vi "KeyboardSimCore.vi"(0 "VI Reference In":refnum<vi>, 1 "Label (VI Title)":string="Default", 11 "error in (no error)":errorcluster) -> (4 "VI Reference Out":refnum<vi>, 15 "error out":errorcluster)   [LabVIEW 2016, in "DronaTest.lvlib"]
uses:
  DronaTest.lvlib
  apis/Stimulus/KeyBoardSimulation/KeyBoardSimulation.vi
  APIs/Assert/AssertControlValue/Equal.vi
  <vilib>/addons/_JKI Toolkits/Caraya/classes/Assert/Assert Not Error.vi
  <vilib>/addons/_JKI Toolkits/Caraya/classes/Test/Test.lvclass
  Drona.lvlib
  <vilib>/addons/_JKI Toolkits/Caraya/classes/Assert/Assert.lvclass
  apis/Stimulus/KeyBoardSimulation/KeyboardSimulation.lvlib
  apis/Assert/AssertControlValue/AssertControlValue.lvlib
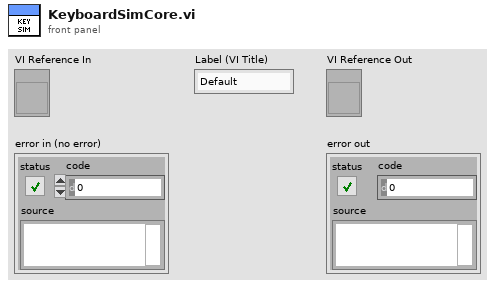
[diagram p1: front panel]
types:
  T1 = enum16{"Typing hello", "Paste from clipboard", "Numeric in range", "Numeric out of range positive", "Numeric out of range negative"}[]
  T2 = cluster{" Key":u8, "Action":enum16{"Press", "Up", "Down"}, "Delay (ms)":u32}[]
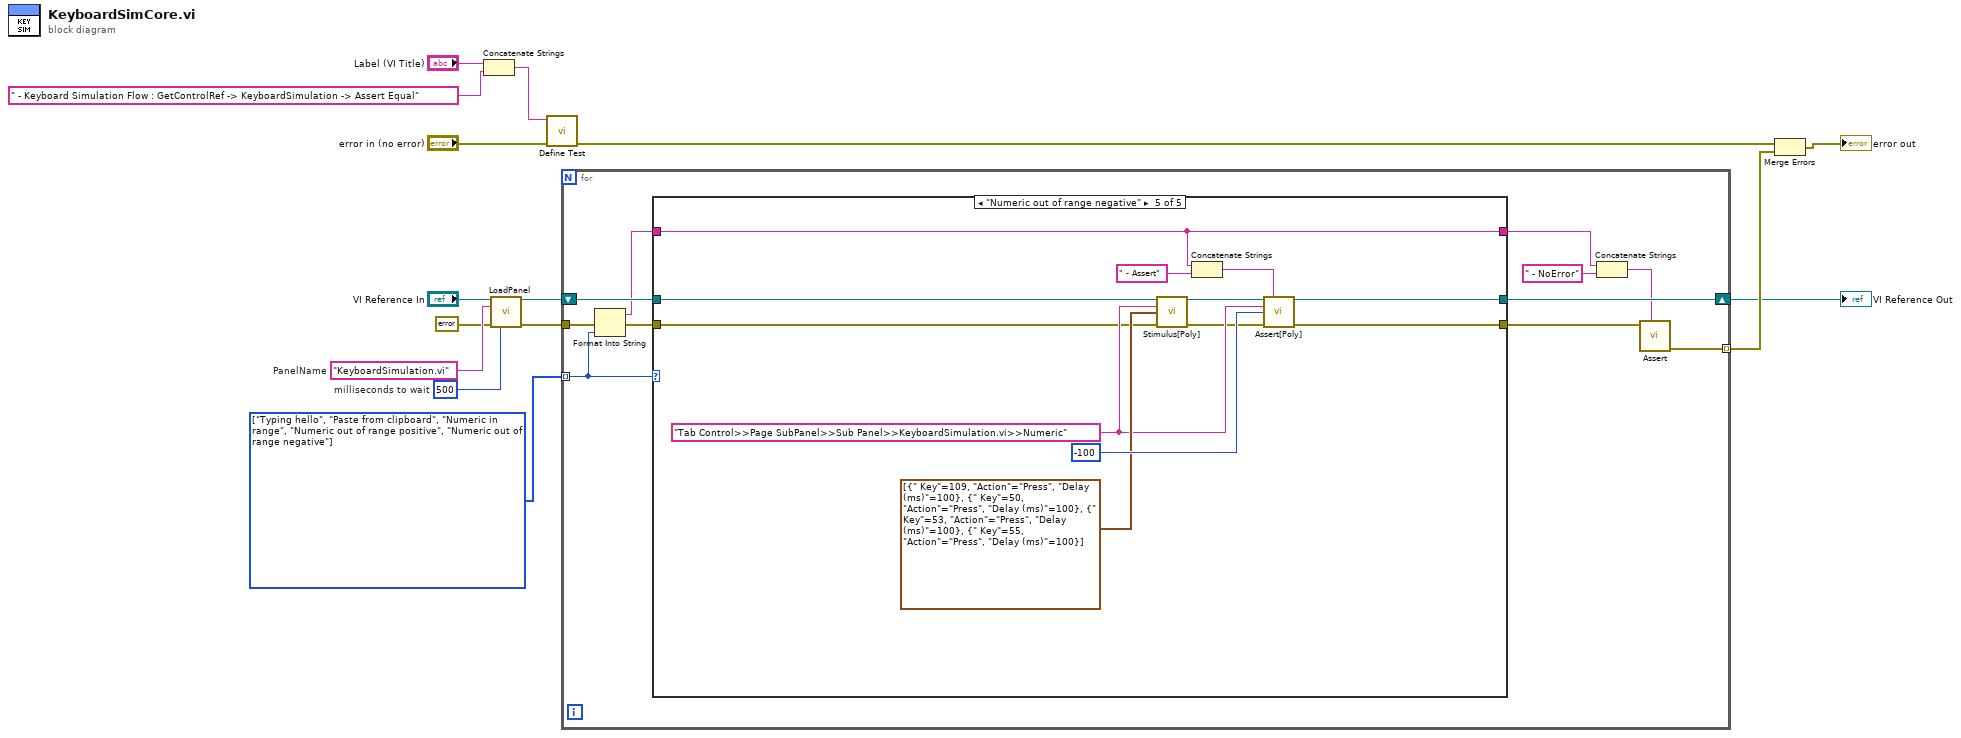
[diagram p0: block diagram]
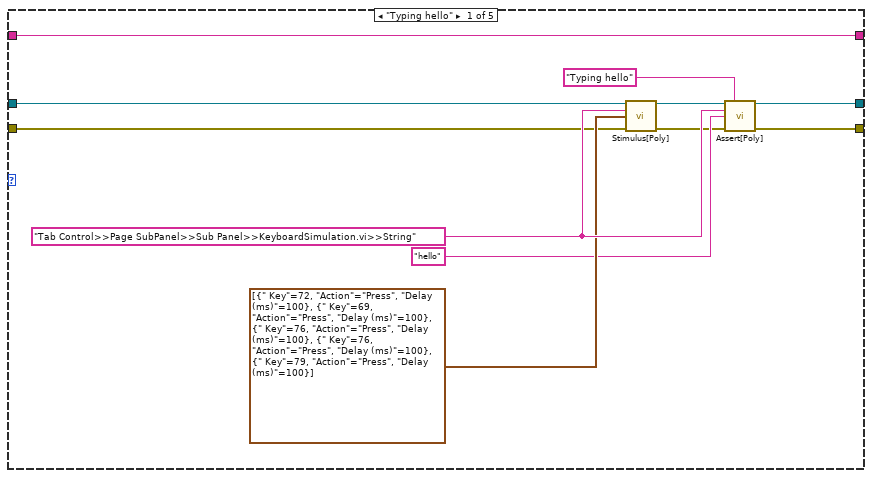
[diagram p2: hidden frame]
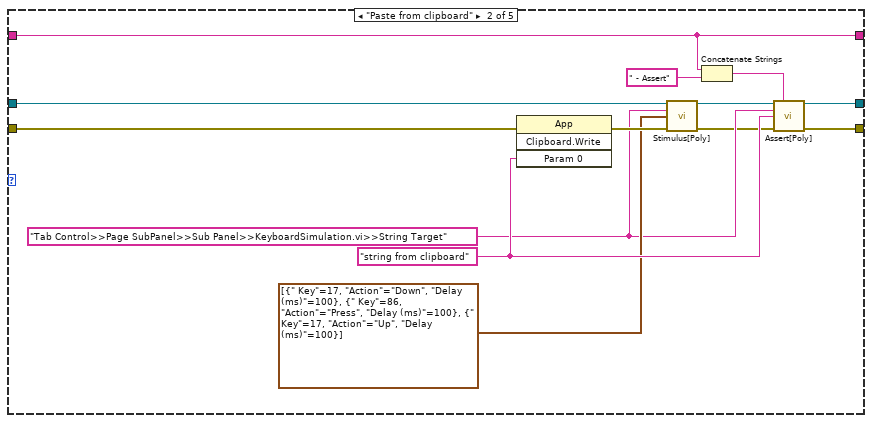
[diagram p3: hidden frame]
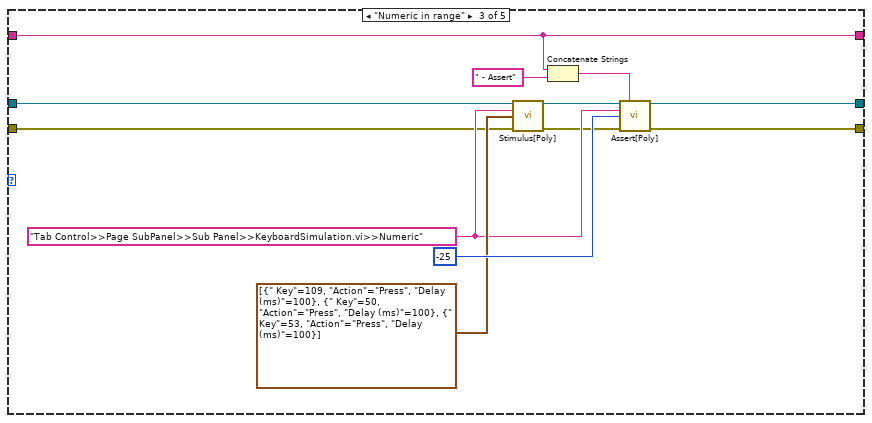
[diagram p4: hidden frame]
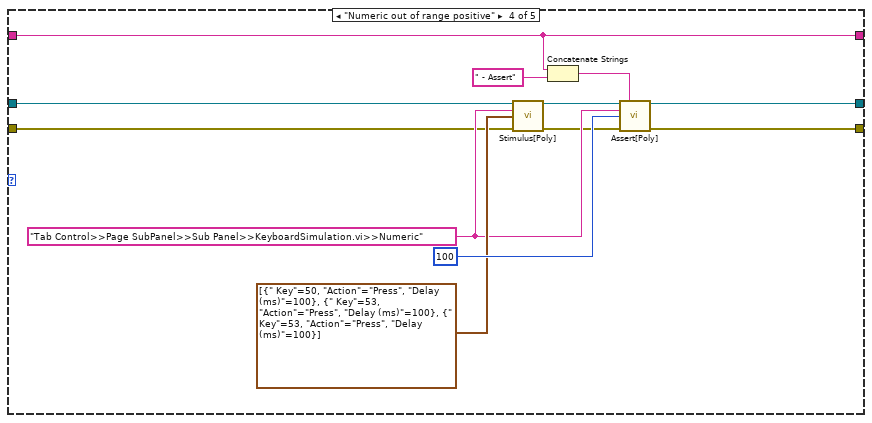
[diagram p5: hidden frame]
diagram:
  w5 = T1 [enum."Typing hello", enum."Paste from clipboard", enum."Numeric in range", enum."Numeric out of range positive", enum."Numeric out of range negative"] items=["Typing hello", "Paste from clipboard", "Numeric in range", "Numeric out of range positive", "Numeric out of range negative"] ("TestCases")
  w6 = u32 500  # milliseconds to wait
  w8 = "KeyboardSimulation.vi"  # PanelName
  n1 = Concatenate Strings("Label (VI Title)", " - Keyboard Simulation Flow : GetControlRef -> KeyboardSimulation -> Assert Equal" ("Label (VI Title)")) -> (w10:string)
  n2 = call "LoadPanel.vi"("VI in"="VI Reference In", "Panel Name"=w8, "error in (no error)"=errorcluster {"status"=FALSE, "code"=0, "source"=""} ("error in"), "milliseconds to wait"=w6) -> ("VI out"=w2:refnum<vi>, "error out"=w4:errorcluster)  [unwired: 10 in]
  n3 = call <vilib>:"Define Test.vi"("error in (no error)"="error in (no error)", "Label (VI Title)"=w10) -> ("error out"=w13:errorcluster)  [unwired: 9 in]
  n4 = for {
    tunnel: w5 -> [w19] mode=indexing
    shift-right: [w25] -> w1
    shift-left: w2 -> [w26]
    tunnel: w4 -> [w24]
    tunnel: [w21] -> w3 mode=indexing
    n5 = Format Into String(error in=w24, w19) -> (resulting string=w18:string, error out=w20:errorcluster)  [unwired: 2 in]
    n6 = case shown="\"Numeric out of range negative\"" w19 {
      tunnel: [w31 w43 w56 w68 w80] -> w22
      tunnel: w26 -> [w30 w41 w54 w66 w78]
      tunnel: [w29 w42 w55 w67 w79] -> w25
      tunnel: w20 -> [w27 w40 w53 w65 w77]
      tunnel: [w28 w38 w51 w63 w75] -> w16
      tunnel: w18 -> [w28 w38 w51 w63 w75]
      frame "Typing hello" {
        w37 = "Tab Control>>Page SubPanel>>Sub Panel>>KeyboardSimulation.vi>>String" ("Control Path")
        n7 = call-poly "Stimulus[Poly].vi"("VI Reference In"=w30, "Control Path"=w37, "Key Array"=T2 [{" Key"=72, "Action"=enum."Press", "Delay (ms)"=100}, {" Key"=69, "Action"=enum."Press", "Delay (ms)"=100}, {" Key"=76, "Action"=enum."Press", "Delay (ms)"=100}, {" Key"=76, "Action"=enum."Press", "Delay (ms)"=100}, {" Key"=79, "Action"=enum."Press", "Delay (ms)"=100}], "error In"=w27) -> ("VI Reference Out"=w33:refnum<vi>, "error IO"=w32:errorcluster)  [unwired: 10 in]
        n8 = call-poly "Assert[Poly].vi"("VI Reference In"=w33, "Label"="Typing hello" ("string"), "Control Path"=w37, "Control Value"="hello" ("Control Path"), "Error In"=w32) -> ("VI Reference Out"=w29:refnum<vi>, "Error Out"=w31:errorcluster)  [unwired: 9 in]
      }
      frame "Paste from clipboard" {
        w50 = "string from clipboard" ("Control Path")
        w47 = "Tab Control>>Page SubPanel>>Sub Panel>>KeyboardSimulation.vi>>String Target" ("Control Path")
        n9 = invoke on="Invoke Node" class="App" method="Clipboard.Write"(error in=w40, "Param 0"=w50) -> (error out=w49:errorcluster)  [unwired: 2 in, 3 out]
        n10 = call-poly "Stimulus[Poly].vi"("VI Reference In"=w41, "Control Path"=w47, "Key Array"=T2 [{" Key"=17, "Action"=enum."Down", "Delay (ms)"=100}, {" Key"=86, "Action"=enum."Press", "Delay (ms)"=100}, {" Key"=17, "Action"=enum."Up", "Delay (ms)"=100}], "error In"=w49) -> ("VI Reference Out"=w45:refnum<vi>, "error IO"=w46:errorcluster)  [unwired: 10 in]
        n11 = Concatenate Strings(w38, " - Assert" ("string")) -> (w39:string)
        n12 = call-poly "Assert[Poly].vi"("VI Reference In"=w45, "Label"=w39, "Control Path"=w47, "Control Value"=w50, "Error In"=w46) -> ("VI Reference Out"=w42:refnum<vi>, "Error Out"=w43:errorcluster)  [unwired: 9 in]
      }
      frame "Numeric in range" {
        w60 = "Tab Control>>Page SubPanel>>Sub Panel>>KeyboardSimulation.vi>>Numeric" ("Control Path")
        n13 = call-poly "Stimulus[Poly].vi"("VI Reference In"=w54, "Control Path"=w60, "Key Array"=T2 [{" Key"=109, "Action"=enum."Press", "Delay (ms)"=100}, {" Key"=50, "Action"=enum."Press", "Delay (ms)"=100}, {" Key"=53, "Action"=enum."Press", "Delay (ms)"=100}], "error In"=w53) -> ("VI Reference Out"=w58:refnum<vi>, "error IO"=w59:errorcluster)  [unwired: 10 in]
        n14 = Concatenate Strings(w51, " - Assert" ("string")) -> (w52:string)
        n15 = call-poly "Assert[Poly].vi"("VI Reference In"=w58, "Label"=w52, "Control Path"=w60, "Control Value"=-25 ("Control Path"), "Error In"=w59) -> ("VI Reference Out"=w55:refnum<vi>, "Error Out"=w56:errorcluster)  [unwired: 9 in]
      }
      frame "Numeric out of range positive" {
        w72 = "Tab Control>>Page SubPanel>>Sub Panel>>KeyboardSimulation.vi>>Numeric" ("Control Path")
        n16 = call-poly "Stimulus[Poly].vi"("VI Reference In"=w66, "Control Path"=w72, "Key Array"=T2 [{" Key"=50, "Action"=enum."Press", "Delay (ms)"=100}, {" Key"=53, "Action"=enum."Press", "Delay (ms)"=100}, {" Key"=53, "Action"=enum."Press", "Delay (ms)"=100}], "error In"=w65) -> ("VI Reference Out"=w70:refnum<vi>, "error IO"=w71:errorcluster)  [unwired: 10 in]
        n17 = Concatenate Strings(w63, " - Assert" ("string")) -> (w64:string)
        n18 = call-poly "Assert[Poly].vi"("VI Reference In"=w70, "Label"=w64, "Control Path"=w72, "Control Value"=100 ("Control Path"), "Error In"=w71) -> ("VI Reference Out"=w67:refnum<vi>, "Error Out"=w68:errorcluster)  [unwired: 9 in]
      }
      frame "Numeric out of range negative" {
        w84 = "Tab Control>>Page SubPanel>>Sub Panel>>KeyboardSimulation.vi>>Numeric" ("Control Path")
        n19 = call-poly "Stimulus[Poly].vi"("VI Reference In"=w78, "Control Path"=w84, "Key Array"=T2 [{" Key"=109, "Action"=enum."Press", "Delay (ms)"=100}, {" Key"=50, "Action"=enum."Press", "Delay (ms)"=100}, {" Key"=53, "Action"=enum."Press", "Delay (ms)"=100}, {" Key"=55, "Action"=enum."Press", "Delay (ms)"=100}], "error In"=w77) -> ("VI Reference Out"=w82:refnum<vi>, "error IO"=w83:errorcluster)  [unwired: 10 in]
        n20 = Concatenate Strings(w75, " - Assert" ("string")) -> (w76:string)
        n21 = call-poly "Assert[Poly].vi"("VI Reference In"=w82, "Label"=w76, "Control Path"=w84, "Control Value"=-100 ("Control Path"), "Error In"=w83) -> ("VI Reference Out"=w79:refnum<vi>, "Error Out"=w80:errorcluster)  [unwired: 9 in]
      }
    }
    n22 = Concatenate Strings(w16, " - NoError" ("string")) -> (w17:string)
    n23 = call-poly <vilib>:"Assert.vi"("Label"=w17, "Not Error?"=w22) -> ("error out"=w21:errorcluster)  [unwired: 9 in]
  }
  "VI Reference Out" <- w1
  n24 = Merge Errors(w13, w3) -> (→"error out":errorcluster)
